vi "DSF.Engine.Builder.Run.vi"(8 "error in (no error)":errorcluster, 10 "Thread Parameters":refnum<class "Thread Parameters.lvclass">, 11 "Builder in":refnum<class "DSF.Engine.Builder.lvclass">) -> (0 "error out":errorcluster, 2 "Builder Interface":refnum<class "DSF.Engine.Interface.Builder.lvclass">, 3 "Builder out":refnum<class "DSF.Engine.Builder.lvclass">)   [LabVIEW 2016, in "DSF.Engine.lvlib" / "DSF.Engine.Builder.lvclass"]
uses:
  DSF.Engine.Builder.lvclass
  Thread Parameters/Thread Parameters.lvclass
  Interface/DSF.Engine.Interface.Builder.lvclass
  DSF.Engine.Builder.lvclass/DSF.Engine.Builder.ctl
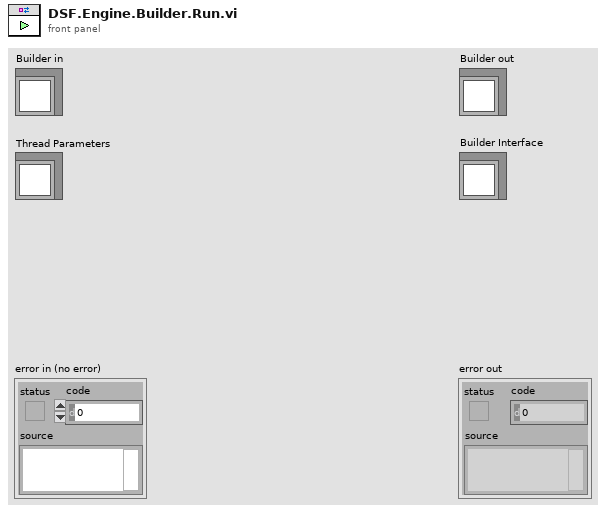
[diagram p1: front panel]
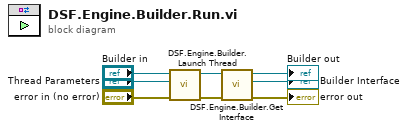
[diagram p0: block diagram]
diagram:
  n1 = call "DSF.Engine.Builder.Launch Thread.vi"("error in (no error)"="error in (no error)", "Thread Parameters"="Thread Parameters", "Builder in"="Builder in") -> ("error out"=→"error out":errorcluster, "Builder out"=w4:refnum<class "DSF.Engine.Builder.lvclass">)  [unwired: 7 in]
  n2 = call "DSF.Engine.Builder.Get Interface.vi"("Builder in"=w4) -> ("Builder Interface"=→"Builder Interface":refnum<class "DSF.Engine.Interface.Builder.lvclass">, "Builder out"=→"Builder out":refnum<class "DSF.Engine.Builder.lvclass">)  [unwired: 9 in]
